vi "WebcamReadandOverlay.vi"() -> ()   [LabVIEW 2015]
panel:
  in  "WebcamFilePath":path
  in  "OverlayText":string
  in  "BasePathToSaveTo":path
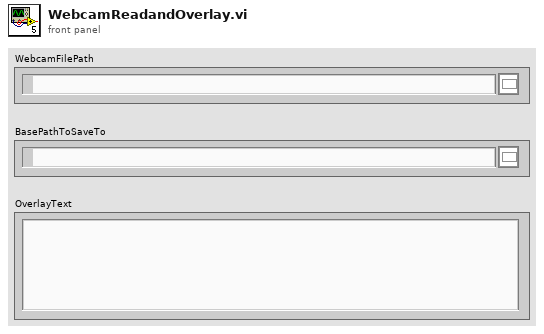
[diagram p1: front panel]
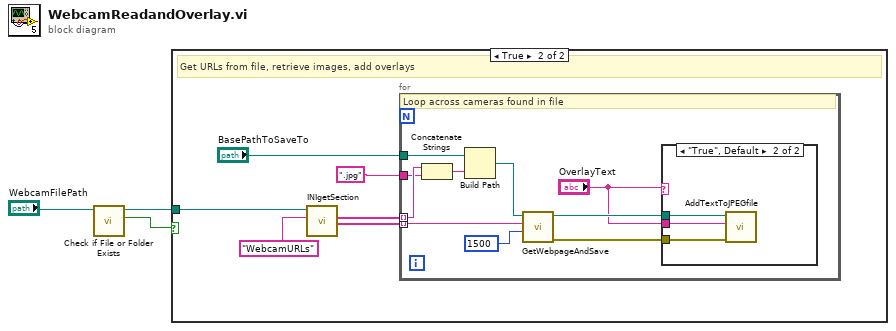
[diagram p0: block diagram]
diagram:
  n1 = call <vilib>:"Check if File or Folder Exists.vi"("path"="WebcamFilePath") -> ("file or folder exists?"=w1:bool, "dup path"=w2:path)  [unwired: 8 in, 1 out]
  n2 = case shown="True" w1 {
    tunnel: w2 -> [_ w4]
    frame False {
      # "No webcam file around here.. do nothing..."
    }
    frame True {
      # "Get URLs from file, retrieve images, add overlays"
      n3 = call "INIgetSection.vi"("SectionName"="WebcamURLs", "INIfilePath"=w4) -> ("SectionValues"=w9:string[], "SectionKeys"=w7:string[])  [unwired: 7 in, 1 out]
      n4 = for {
        tunnel: w9 -> [w17] mode=indexing
        tunnel: "BasePathToSaveTo" -> [w15]
        tunnel: w7 -> [w14] mode=indexing
        tunnel: ".jpg" -> [w12]
        # "Loop across cameras found in file"
        n5 = Concatenate Strings(w14, w12) -> (w13:string)
        n6 = Build Path(base path=w15, name or relative path=w13) -> (appended path=w16:path)
        n7 = call "GetWebpageAndSave.vi"("timeout (ms)"=1500, "url"=w17, "pathIn"=w16) -> ("error out"=w18:errorcluster, "pathOut"=w19:path)  [unwired: 7 in]
        n8 = case shown="\"True\", Default" "OverlayText" {
          tunnel: w19 -> [_ w22]
          tunnel: w18 -> [_ w21]
          tunnel: "OverlayText" -> [_ w20]
          frame "\u0000" {
          }
          frame "True", Default {
            n9 = call "AddTextToJPEGfile.vi"("error in (no error)"=w21, "text"=w20, "pathIn"=w22) -> ()  [unwired: 8 in, 1 out]
          }
        }
      }
    }
  }
